vi "Scale Output L3G4200D.vi"(9 "Byte1":u8, 11 "Byte0":u8) -> (3 "Rotation Rate (mdps)":dbl)   [LabVIEW 2015]
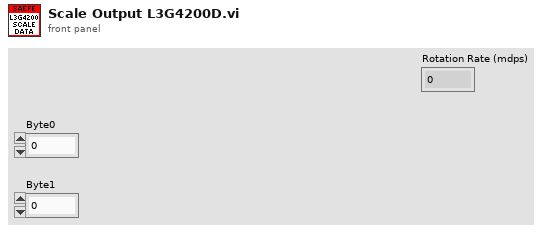
[diagram p1: front panel]
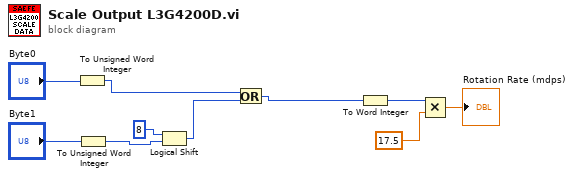
[diagram p0: block diagram]
diagram:
  n1 = To Unsigned Word Integer(number="Byte0") -> (unsigned 16bit integer=w6:u16)
  n2 = To Unsigned Word Integer(number="Byte1") -> (unsigned 16bit integer=w8:u16)
  n3 = Logical Shift(y=i16 8, x=w8) -> (x << y=w5:u16)
  n4 = Or(x=w6, y=w5) -> (x .or. y?=w1:u16)
  n5 = To Word Integer(number=w1) -> (16bit integer=w4:i16)
  n6 = Multiply(x=w4, y=17.5) -> (x*y=→"Rotation Rate (mdps)":dbl)
